vi "Open Hardware.vi"(8 "error in (no error)":errorcluster, 11 "Instrument in":refnum<class "Instrument.lvclass">) -> (0 "error out":errorcluster, 3 "Instrument out":refnum<class "Instrument.lvclass">)   [LabVIEW 2019, in "Instrument.lvlib" / "Instrument.lvclass"]
doc: "Override to <b>open</b> a connection to your instrument."
uses:
  Instrument.lvclass
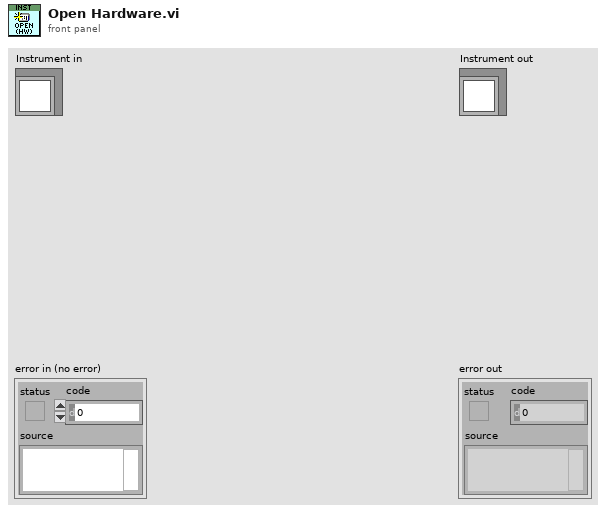
[diagram p1: front panel]
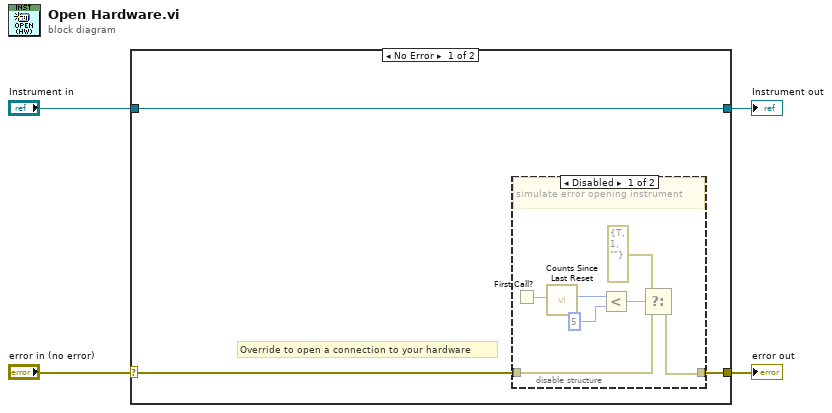
[diagram p0: block diagram]
diagram:
  n1 = case shown="No Error" "error in (no error)" {
    selector: "error in (no error)" -> [w6 w17]
    tunnel: [w5 w17] -> w3
    tunnel: [w7 w16] -> w1
    tunnel: "Instrument in" -> [w7 w16]
    frame No Error {
      # "Override to open a connection to your hardware"
      n2 = disable-structure shown="Disabled" {
        disable-tunnel: w6 -> [w13 w15]
        disable-tunnel: [w12 w15] -> w5
        frame Disabled {
          # "simulate error opening instrument"
          n3 = First Call?() -> (First Call?: T/F=w9:bool)
          n4 = call "Counts Since Last Reset.vi"("Reset (F)"=w9) -> ("counter"=w8:u32)  [unwired: 5 in, 1 out]
          n5 = Less?(x=w8, y=u32 5 ("x")) -> (x < y?=w14:bool)
          n6 = Select(t=errorcluster {"status"=TRUE, "code"=1, "source"=""}, s=w14, f=w13) -> (s? t:f=w12:errorcluster)
        }
        frame Enabled {
        }
      }
    }
    frame Error {
    }
  }
  "error out" <- w3
  "Instrument out" <- w1
